vi "sub_SDR_mimo_tx.vi"(6 "Init Tx Buffer":bool, 7 "System options":T1, 10 "Packets":string[](array[string])) -> (0 "Link occupation [%]":dbl, 1 "Tx Buffer size":i32, 2 "Data out (2D)":cdb[][](array[numeric]), 3 "Ok?":bool)   [LabVIEW 2012]
panel:
  out "size(s)":i32
  out "Payload Length (char)":i32
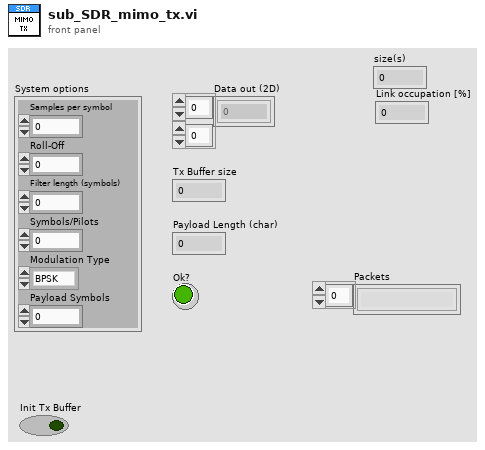
[diagram p1: front panel]
types:
  T1 = cluster{"Samples per symbol":i32, "Roll-Off":dbl, "Filter length (symbols)":i32, "Symbols/Pilots":i32, "Modulation Type":enum16{"BPSK", "4-QAM", "16-QAM", "64-QAM"}, "Payload Symbols":i32}
  T2 = cluster{"Samples per symbol":i32, "Roll-Off":dbl, "Filter length (symbols)":i32}
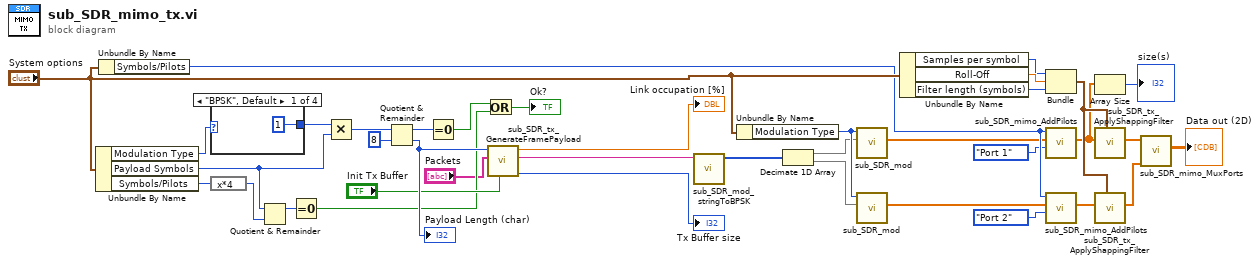
[diagram p0: block diagram]
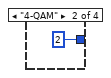
[diagram p2: hidden frame]
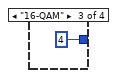
[diagram p3: hidden frame]
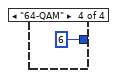
[diagram p4: hidden frame]
diagram:
  n1 = Unbundle By Name("System options") -> ("Modulation Type"=w33:enum16{"BPSK", "4-QAM", "16-QAM", "64-QAM"}, "Payload Symbols"=w11:i32, "Symbols/Pilots"=w12:i32)
  n2 = Unbundle By Name("System options") -> ("Symbols/Pilots"=w23:i32)
  n3 = case shown="\"BPSK\", Default" w33 {
    tunnel: [1 2 4 6] -> w34
    frame "BPSK", Default {
    }
    frame "4-QAM" {
    }
    frame "16-QAM" {
    }
    frame "64-QAM" {
    }
  }
  n4 = expression code="x*4"(w12) -> (w10:i32)
  n5 = Quotient & Remainder(x=w11, y=w10) -> (x-y*floor(x/y)=w9:i32)  [unwired: 1 out]
  n6 = Equal To 0?(x=w9) -> (x = 0?=w6:bool)
  n7 = Multiply(x=w34, y=w11) -> (x*y=w36:i32)
  n8 = Quotient & Remainder(x=w36, y=8) -> (x-y*floor(x/y)=w38:i32, floor(x/y)=w37:i32)
  "Payload Length (char)" <- w37
  n9 = Equal To 0?(x=w38) -> (x = 0?=w7:bool)
  n10 = Or(x=w7, y=w6) -> (x .or. y?=→"Ok?":bool)
  n11 = call "sub_SDR_tx_GenerateFramePayload.vi"("Init?"="Init Tx Buffer", "Packets"="Packets", "Payload Length"=w37) -> ("Buffer Length"=→"Tx Buffer size":i32, "Payload String"=w15:string, "Link occupation [%]"=→"Link occupation [%]":dbl)  [unwired: 6 in]
  n12 = call "sub_SDR_mod_stringToBPSK.vi"("Input String"=w15) -> ("Array"=w16:i16[])  [unwired: 10 in]
  n13 = Unbundle By Name("System options") -> ("Modulation Type"=w19:enum16{"BPSK", "4-QAM", "16-QAM", "64-QAM"})
  n14 = Decimate 1D Array ("Deinterleave bits")(w16) -> (w17:i16[], w18:i16[])
  n15 = call "sub_SDR_mod.vi"("Array"=w17, "Modulation Type"=w19) -> ("Array out"=w5:cdb[])  [unwired: 9 in]
  n16 = call "sub_SDR_mod.vi"("Array"=w18, "Modulation Type"=w19) -> ("Array out"=w21:cdb[])  [unwired: 9 in]
  n17 = Unbundle By Name("System options") -> ("Samples per symbol"=w28:i32, "Roll-Off"=w29:dbl, "Filter length (symbols)"=w30:i32)
  n18 = Bundle("Samples per symbol"=w28, "Roll-Off"=w29, "Filter length (symbols)"=w30) -> (w31:T2)  [unwired: 1 in]
  n19 = call "sub_SDR_mimo_AddPilots.vi"("Port"=enum16{"Port 1", "Port 2"}."Port 1", "Array in"=w5, "Symbols/Pilots"=w23) -> ("Array Out"=w3:cdb[])  [unwired: 8 in]
  n20 = call "sub_SDR_mimo_AddPilots.vi"("Port"=enum16{"Port 1", "Port 2"}."Port 2", "Array in"=w21, "Symbols/Pilots"=w23) -> ("Array Out"=w24:cdb[])  [unwired: 8 in]
  n21 = Array Size(array=w3) -> (size(s)=→"size(s)":i32)
  n22 = call "sub_SDR_tx_ApplyShappingFilter.vi"("Filter Options"=w31, "Data Symbols"=w3) -> ("Shaped symbols"=w26:cdb[])  [unwired: 9 in]
  n23 = call "sub_SDR_tx_ApplyShappingFilter.vi"("Filter Options"=w31, "Data Symbols"=w24) -> ("Shaped symbols"=w27:cdb[])  [unwired: 9 in]
  n24 = call "sub_SDR_mimo_MuxPorts.vi"("Port 2 in"=w27, "Port 1 in"=w26) -> ("Data out (2D)"=→"Data out (2D)":cdb[][])  [unwired: 9 in]
